vi "Nests Destroyed.vi"(11 "Self Actor in":refnum<class "Self Actor.lvclass">) -> (1 "Nest Msg Q DVRs":set{refnum<data-value>}(c389), 2 "Nests Destroyed?":bool)   [LabVIEW 2021, in "LVCAM.lvlib" / "Self Actor.lvclass"]
uses:
  Self Actor.lvclass
  Msg Strategy/Msg Strategy.lvclass
  Self Actor.lvclass/Self Actor.ctl
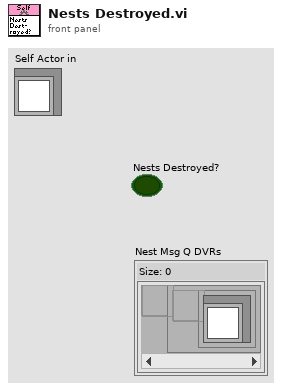
[diagram p1: front panel]
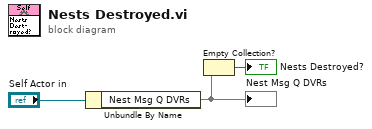
[diagram p0: block diagram]
diagram:
  n1 = Unbundle By Name("Self Actor in") -> ("Nest Msg Q DVRs"=w2:set{refnum<data-value>})
  "Nest Msg Q DVRs" <- w2
  n2 = Empty Collection?(1:w2) -> (0:→"Nests Destroyed?":bool)
